vi "Update Object by Type.vi"(7 "Overwrite? (F)":bool, 8 "error in (no error)":errorcluster, 10 "Object":refnum<class>, 11 "Processing in":refnum<class "Processing.lvclass">) -> (0 "error out":errorcluster, 3 "Processing out":refnum<class "Processing.lvclass">)   [LabVIEW 2020, in "HTTP Server.lvlib" / "Processing.lvclass"]
uses:
  Processing.lvclass
  Values/Values.lvclass
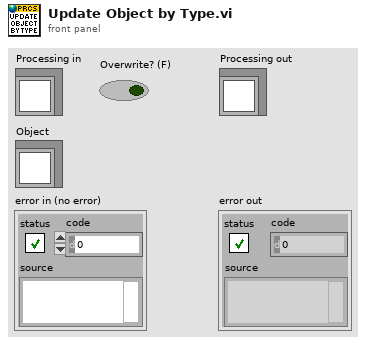
[diagram p1: front panel]
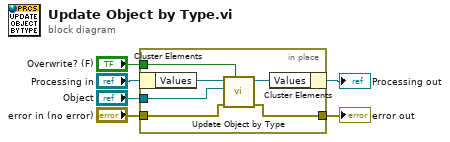
[diagram p0: block diagram]
diagram:
  n1 = in-place {
    in-place-border: "Overwrite? (F)" -> [w11]
    in-place-border: "Object" -> [w10]
    in-place-border: "error in (no error)" -> [w8]
    in-place-border: [w7] -> w2
    n2 = in-place-cluster #1("Processing in") -> ("Values"=w12:refnum<class "Values.lvclass">)
    n3 = call "Update Object by Type.vi"("Overwrite? (F)"=w11, "error in (no error)"=w8, "Object"=w10, "Values in"=w12) -> ("error out"=w7:errorcluster, "Values out"=w9:refnum<class "Values.lvclass">)  [unwired: 6 in]
    n4 = in-place-cluster #1("Values"=w9) -> (→"Processing out":refnum<class "Processing.lvclass">)
  }
  "error out" <- w2
